vi "GetDateTimeString.vi"(2 "前导字符(F:无)":bool, 4 "time stamp":timestamp) -> (0 "YYYYMMDD":string, 1 "date/time string":string)   [LabVIEW 2018]
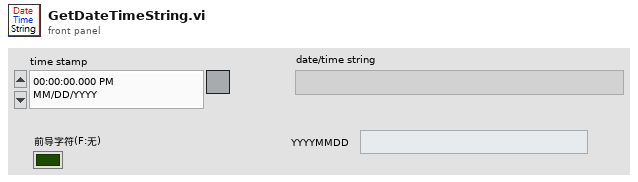
[diagram p1: front panel]
types:
  T1 = typedef "LVDateTimeRec.ctl" = cluster{"fractional second":dbl, "second":i32, "minute":i32, "hour":i32, "day of month":i32, "month":i32, "year":i32, "day of week":i32, "day of year":i32, "DST":i32}
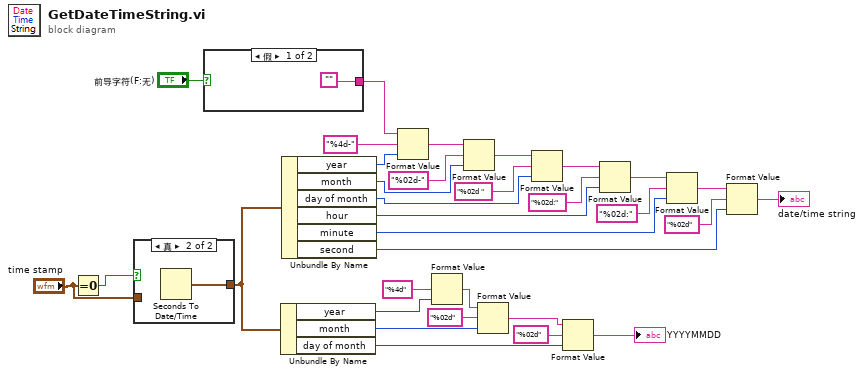
[diagram p0: block diagram]
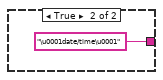
[diagram p2: hidden frame]
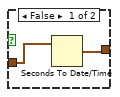
[diagram p3: hidden frame]
diagram:
  n1 = Equal To 0?(x="time stamp") -> (x = 0?=w13:bool)
  n2 = case shown="真" w13 {
    tunnel: [w33 w35] -> w10
    tunnel: "time stamp" -> [w34 _]
    frame False {
      n3 = Seconds To Date/Time(time stamp (now)=w34) -> (date time rec=w33:T1)  [unwired: 1 in]
    }
    frame True {
      n4 = Seconds To Date/Time() -> (date time rec=w35:T1)  [unwired: 2 in]
    }
  }
  n5 = case shown="假" "前导字符(F:无)" {
    tunnel: ["" "\u0001date/time\u0001" ("string (\"\")")] -> w14
    frame False {
    }
    frame True {
    }
  }
  n6 = Unbundle By Name(w10) -> ("year"=w8:i32, "month"=w7:i32, "day of month"=w4:i32)
  n7 = Unbundle By Name(w10) -> ("year"=w20:i32, "month"=w19:i32, "day of month"=w18:i32, "hour"=w32:i32, "minute"=w29:i32, "second"=w28:i32)
  n8 = Format Value(string ("")=w14, format string="%4d-", value (0)=w20) -> (output string=w23:string)
  n9 = Format Value(format string="%4d", value (0)=w8) -> (output string=w6:string)  [unwired: 1 in]
  n10 = Format Value(string ("")=w23, format string="%02d-", value (0)=w19) -> (output string=w22:string)
  n11 = Format Value(string ("")=w6, format string="%02d", value (0)=w7) -> (output string=w3:string)
  n12 = Format Value(string ("")=w22, format string="%02d ", value (0)=w18) -> (output string=w21:string)
  n13 = Format Value(string ("")=w3, format string="%02d", value (0)=w4) -> (output string=→"YYYYMMDD":string)
  n14 = Format Value(string ("")=w21, format string="%02d:", value (0)=w32) -> (output string=w31:string)
  n15 = Format Value(string ("")=w31, format string="%02d:", value (0)=w29) -> (output string=w30:string)
  n16 = Format Value(string ("")=w30, format string="%02d", value (0)=w28) -> (output string=→"date/time string":string)
